vi "Write Schedule.vi"(8 "error in (no error)":errorcluster, 10 "Schedule":T1, 11 "Parameters in":refnum<class "Parameters.lvclass">) -> (0 "error out":errorcluster, 3 "Parameters out":refnum<class "Parameters.lvclass">)   [LabVIEW 2020, in "Parameters.lvclass"]
uses:
  Parameters.lvclass
  Typedefs/Tosca-Schedule.ctl
  Typedefs/Tosca-Sequence Order.ctl
  Typedefs/Tosca-Parameter Family.ctl
  Typedefs/Tosca-Parameter Table Element.ctl
  Typedefs/Tosca-Parameter Dimension.ctl
  Parameters.lvclass/Parameters.ctl
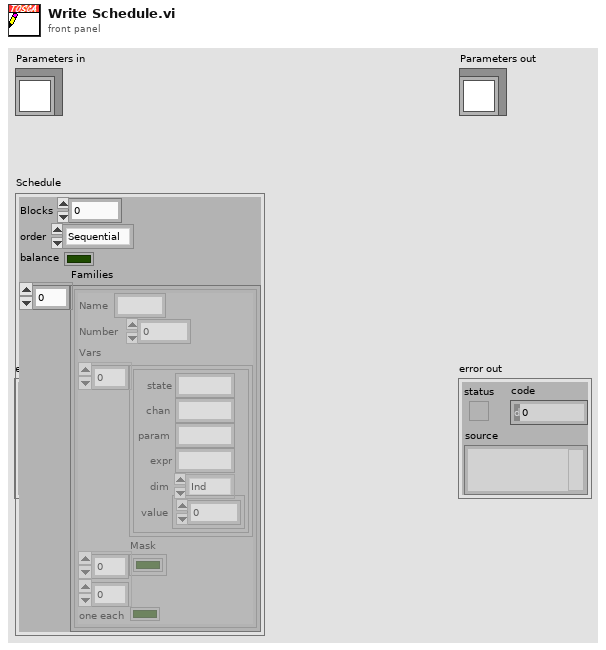
[diagram p1: front panel]
types:
  T1 = typedef "Tosca-Schedule.ctl" = cluster{"Blocks":i32, "order":T2, "balance":bool, "Families":T3[]}
  T2 = typedef "Tosca-Sequence Order.ctl" = enum16{"Sequential", "Alternate", "Randomize", "Random group"}
  T3 = typedef "Tosca-Parameter Family.ctl" = cluster{"Name":string, "Number":i32, "Vars":T4[], "Mask":bool[][], "one each":bool}
  T4 = typedef "Tosca-Parameter Table Element.ctl" = cluster{"state":string, "chan":string, "param":string, "expr":string, "dim":T5, "value":dbl[]}
  T5 = typedef "Tosca-Parameter Dimension.ctl" = enum16{"Ind", "X", "Y"}
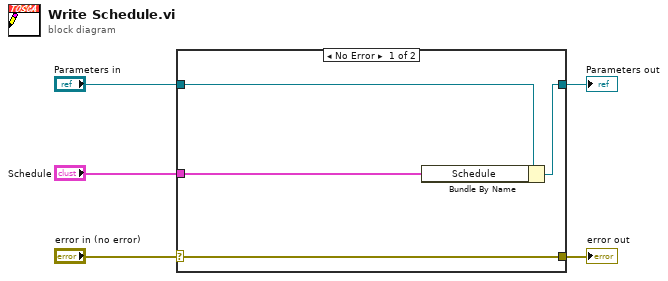
[diagram p0: block diagram]
diagram:
  n1 = case shown="No Error" "error in (no error)" {
    selector: "error in (no error)" -> [w9 w10]
    tunnel: [w9 w10] -> w4
    tunnel: [w7 w11] -> w2
    tunnel: "Parameters in" -> [w8 w11]
    tunnel: "Schedule" -> [w6 _]
    frame No Error {
      n2 = Bundle By Name(cluster=w8, "Schedule"=w6) -> (w7:refnum<class "Parameters.lvclass">)
    }
    frame Error {
    }
  }
  "error out" <- w4
  "Parameters out" <- w2
